vi "NULLcharacterKILLERarray.vi"(1 "Input Array":string[](array[string]), 2 "Null position":enum16{"First", "Second"}(ring)) -> (0 "Cleaned Array":string[](array[string]))   [LabVIEW 2019]
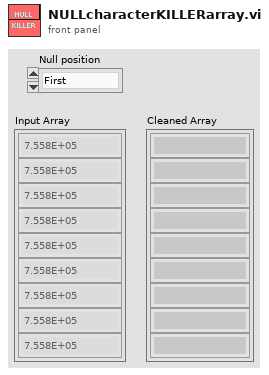
[diagram p1: front panel]
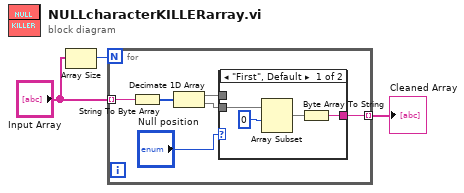
[diagram p0: block diagram]
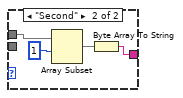
[diagram p2: hidden frame]
diagram:
  n1 = Array Size(array="Input Array") -> (size(s)=w2:i32)
  n2 = for {
    N: w2 -> [_]
    tunnel: "Input Array" -> [w7] mode=indexing
    tunnel: [w4] -> w1 mode=indexing
    n3 = String To Byte Array(string=w7) -> (unsigned byte array=w9:u8[])
    n4 = Decimate 1D Array(w9) -> (w5:u8[], w8:u8[])
    n5 = case shown="\"First\", Default" "Null position" {
      tunnel: [w12 w16] -> w4
      tunnel: w8 -> [w11 _]
      tunnel: w5 -> [_ w15]
      frame "First", Default {
        n6 = Array Subset(array=w11, index=0) -> (w13:u8[])  [unwired: 1 in]
        n7 = Byte Array To String(unsigned byte array=w13) -> (string=w12:string)
      }
      frame "Second" {
        n8 = Array Subset(array=w15, index=1) -> (w17:u8[])  [unwired: 1 in]
        n9 = Byte Array To String(unsigned byte array=w17) -> (string=w16:string)
      }
    }
  }
  "Cleaned Array" <- w1
